vi "subDFD_LPth Norm Design Example Data.vi"(0 "Example Idx":i32=4) -> (1 "Spec":T2={"pole radius constraint"=0.0, "filter type"=enum."Symmetric", "order"={"num"=6, "den"=6}, "band specs"=[{"frequency point"=[{"frequency"=0.0, "magnitude"=1.0, "weight"=1.0, "phase"=0.0}, {"frequency"=0.25, "magnitude"=1.0, "weight"=1.0, "phase"=0.0}]}, {"frequency point"=[{"frequency"=0.3, "magnitude"=0.0, "weight"=1.0, "phase"=0.0}, {"frequency"=0.5, "magnitude"=0.0, "weight"=1.0, "phase"=0.0}]}], "group delay"=2.0, "fs [Hz]"=1.0, "p (128) 2"=12}, 2 "description":string="Designs an IIR lowpass filter without setting the pole radius constraint. To learn more about this design, switch to the Zero-Pole Plot page to verify that there is a pole very close to the unit circle. Switch to the Magnitude Response page to check the spike at the edge of the passband.")   [LabVIEW 2023]
uses:
  <vilib>/addons/Digital Filter Design/_LpNorm.llb/dfd_Lp Norm Filter Type.ctl
  <vilib>/addons/Digital Filter Design/NI_DigFilterLicensed.lvlib
panel:
  in  "Example Descriptions":string[](array[string])=["Designs a linear phase FIR filter by L2 norm criterion. To learn more about this design, switch to the Phase Response page to check the linear phase property of the designed filter. Switch to the Group Delay page to check the constant values in the passband. Switch to the Specifications page to verify that the group delay value equals half of the numerator order.", "Designs a linear phase FIR filter by L4 norm criterion. To learn more about this design, switch to the Phase Response page to check the linear phase property of the designed filter. Switch to the Group Delay page to check the constant values in the passband. Switch to the Specifications page to verify that the group delay value equals half of the numerator order.", "Designs a linear phase FIR filter by L128 norm (almost L inf norm) criterion. To learn more about this design, switch to the Phase Response page to check the linear phase property of the designed filter. Switch to the Group Delay page to check the constant values in the passband. Switch to the Magnitude Response page to check the equal-ripple property in the passband and stopband. Switch to the Specifications page to verify that the group delay value equals half of the numerator order.", "Designs an approximately linear phase FIR filter by L128 norm (almost L inf norm) criterion. To learn more about this design, switch to the Group Delay page to check the nonconstant values in the passband. Switch to the Specifications page to verify that the group delay value is smaller than half of the numerator order.", "Designs an IIR lowpass filter without setting the pole radius constraint. To learn more about this design, switch to the Pole-Zero Plot page to verify that there is a pole very close to the unit circle. Switch to the Magnitude Response page to check the spike at the edge of the passband.", "Designs an IIR lowpass filter with a pole radius constraint. To learn more about this design, switch to the Pole-Zero Plot page to verify that all the poles are inside the unit circle with the constrained radius. Switch to the Magnitude Response page to verify that there is no spike at the edge of the passband.", "Designs a minimum phase lowpass IIR filter without a radius constraint. Unlike previous examples, which are essentially complex approximation, the minimum phase design is magnitude approximation only. The designed filter achieves a much smaller passband ripple as well as a greater stopband attenuation, as shown on the filter magnitude response graph."]
  in  "Example Settings":T3(array[cluster])=[{"pole radius constraint"=0.9999, "filter type"=enum."Symmetric", "order"={"num"=22, "den"=0}, "band specs"=[{"frequency point"=[{"frequency"=0.0, "magnitude"=1.0, "weight"=1.0, "phase"=0.0}, {"frequency"=0.2, "magnitude"=1.0, "weight"=1.0, "phase"=0.0}]}, {"frequency point"=[{"frequency"=0.3, "magnitude"=0.0, "weight"=1.0, "phase"=0.0}, {"frequency"=0.5, "magnitude"=0.0, "weight"=1.0, "phase"=0.0}]}], "group delay"=11.0, "fs [Hz]"=1.0, "p (128) 2"=2}, {"pole radius constraint"=0.9999, "filter type"=enum."Symmetric", "order"={"num"=22, "den"=0}, "band specs"=[{"frequency point"=[{"frequency"=0.0, "magnitude"=1.0, "weight"=1.0, "phase"=0.0}, {"frequency"=0.2, "magnitude"=1.0, "weight"=1.0, "phase"=0.0}]}, {"frequency point"=[{"frequency"=0.3, "magnitude"=0.0, "weight"=1.0, "phase"=0.0}, {"frequency"=0.5, "magnitude"=0.0, "weight"=1.0, "phase"=0.0}]}], "group delay"=11.0, "fs [Hz]"=1.0, "p (128) 2"=4}, {"pole radius constraint"=0.9999, "filter type"=enum."Symmetric", "order"={"num"=22, "den"=0}, "band specs"=[{"frequency point"=[{"frequency"=0.0, "magnitude"=1.0, "weight"=1.0, "phase"=0.0}, {"frequency"=0.2, "magnitude"=1.0, "weight"=1.0, "phase"=0.0}]}, {"frequency point"=[{"frequency"=0.3, "magnitude"=0.0, "weight"=1.0, "phase"=0.0}, {"frequency"=0.5, "magnitude"=0.0, "weight"=1.0, "phase"=0.0}]}], "group delay"=11.0, "fs [Hz]"=1.0, "p (128) 2"=128}, {"pole radius constraint"=0.9999, "filter type"=enum."Symmetric", "order"={"num"=22, "den"=0}, "band specs"=[{"frequency point"=[{"frequency"=0.0, "magnitude"=1.0, "weight"=1.0, "phase"=0.0}, {"frequency"=0.2, "magnitude"=1.0, "weight"=1.0, "phase"=0.0}]}, {"frequency point"=[{"frequency"=0.3, "magnitude"=0.0, "weight"=1.0, "phase"=0.0}, {"frequency"=0.5, "magnitude"=0.0, "weight"=1.0, "phase"=0.0}]}], "group delay"=9.0, "fs [Hz]"=1.0, "p (128) 2"=128}, {"pole radius constraint"=0.0, "filter type"=enum."Symmetric", "order"={"num"=6, "den"=6}, "band specs"=[{"frequency point"=[{"frequency"=0.0, "magnitude"=1.0, "weight"=1.0, "phase"=0.0}, {"frequency"=0.25, "magnitude"=1.0, "weight"=1.0, "phase"=0.0}]}, {"frequency point"=[{"frequency"=0.3, "magnitude"=0.0, "weight"=1.0, "phase"=0.0}, {"frequency"=0.5, "magnitude"=0.0, "weight"=1.0, "phase"=0.0}]}], "group delay"=2.0, "fs [Hz]"=1.0, "p (128) 2"=12}, {"pole radius constraint"=0.9, "filter type"=enum."Symmetric", "order"={"num"=6, "den"=6}, "band specs"=[{"frequency point"=[{"frequency"=0.0, "magnitude"=1.0, "weight"=1.0, "phase"=0.0}, {"frequency"=0.25, "magnitude"=1.0, "weight"=1.0, "phase"=0.0}]}, {"frequency point"=[{"frequency"=0.3, "magnitude"=0.0, "weight"=1.0, "phase"=0.0}, {"frequency"=0.5, "magnitude"=0.0, "weight"=1.0, "phase"=0.0}]}], "group delay"=2.0, "fs [Hz]"=1.0, "p (128) 2"=12}, {"pole radius constraint"=0.0, "filter type"=enum."Minimum Phase", "order"={"num"=6, "den"=6}, "band specs"=[{"frequency point"=[{"frequency"=0.0, "magnitude"=1.0, "weight"=1.0, "phase"=0.0}, {"frequency"=0.25, "magnitude"=1.0, "weight"=1.0, "phase"=0.0}]}, {"frequency point"=[{"frequency"=0.3, "magnitude"=0.0, "weight"=1.0, "phase"=0.0}, {"frequency"=0.5, "magnitude"=0.0, "weight"=1.0, "phase"=0.0}]}], "group delay"=0.0, "fs [Hz]"=1.0, "p (128) 2"=128}] {"pole radius constraint" min=0.0; "fs [Hz]" format="%.2f"; "band specs"."frequency point"."weight" format="%.2f"}
  # "freq"
  # "magnitude"
  # "weight"
  # "phase"
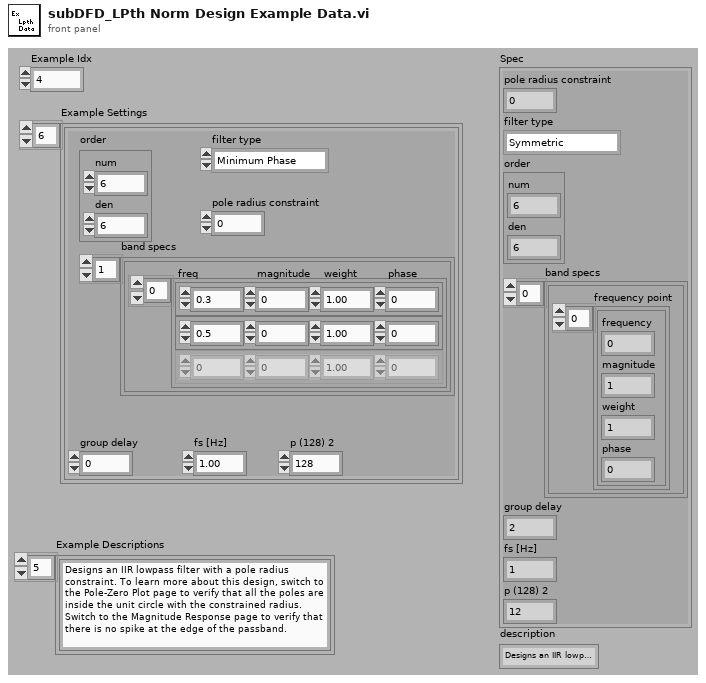
[diagram p1: front panel]
types:
  T1 = typedef "NI_DigFilterLicensed.lvlib/dfd_Lp Norm Filter Type.ctl" = enum16{"Symmetric", "Antisymmetric", "Differentiator", "Hilbert", "Minimum Phase", "Maximum Phase"}
  T2 = cluster{"pole radius constraint":dbl, "filter type":T1, "order":cluster{"num":i32, "den":i32}, "band specs":cluster{"frequency point":cluster{"frequency":dbl, "magnitude":dbl, "weight":dbl, "phase":dbl}[]}[], "group delay":dbl, "fs [Hz]":dbl, "p (128) 2":i32}
  T3 = cluster{"pole radius constraint":dbl, "filter type":T1, "order":cluster{"num":i32, "den":i32}, "band specs":cluster{"frequency point":cluster{"frequency":dbl, "magnitude":dbl, "weight":dbl, "phase":dbl}[]}[], "group delay":dbl, "fs [Hz]":dbl, "p (128) 2":i32}[]
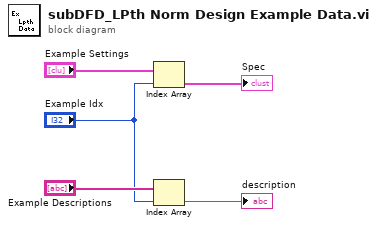
[diagram p0: block diagram]
diagram:
  n1 = Index Array(array="Example Settings", index="Example Idx") -> (element=→"Spec":T2)
  n2 = Index Array(array="Example Descriptions", index="Example Idx") -> (element=→"description":string)
